vi "GrubbsTest_-_kopia.vi"() -> ()   [LabVIEW 2013]
uses:
  <vilib>/Analysis/NI_AALBase.lvlib
  <vilib>/Utility/file.llb/Read From Spreadsheet File (DBL).vi
panel:
  out "СКО":dbl
  out "Среднее":dbl
  out "Обработанные":dbl[](graph)
  out "Исходные":dbl[](graph)
  out "Промахи":dbl[](array[numeric])
  in  "Значимость":dbl
  in  "Path":path
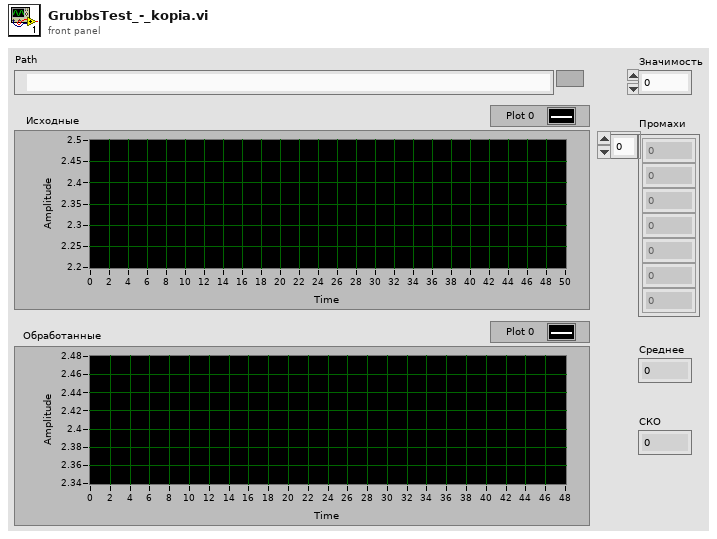
[diagram p1: front panel]
types:
  T1 = enum16{"Init", "GradeCount", "MissChecks", "fin"}
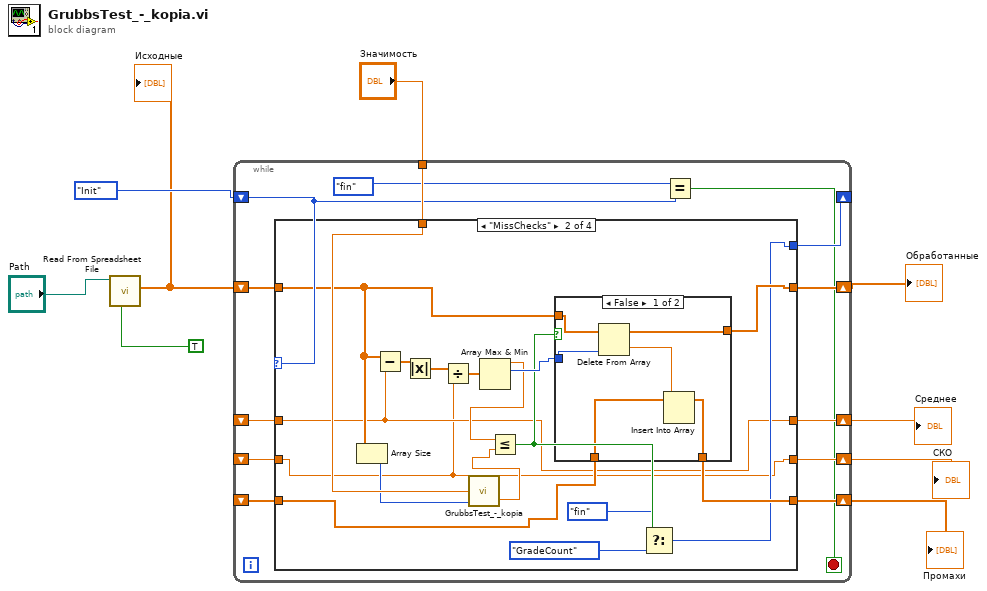
[diagram p0: block diagram]
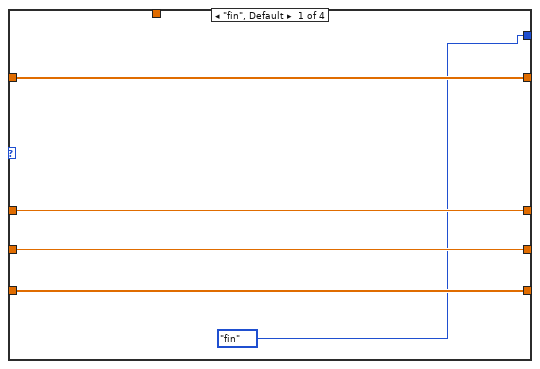
[diagram p2: hidden frame]
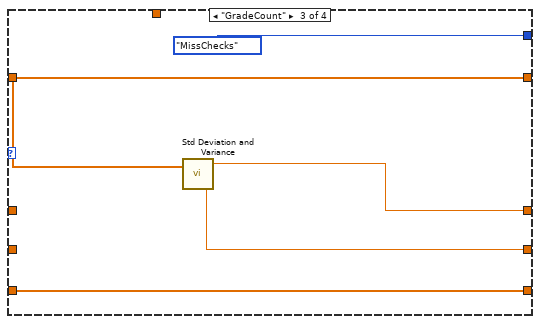
[diagram p4: hidden frame]
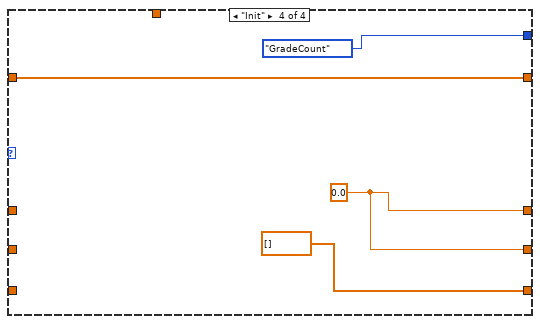
[diagram p5: hidden frame]
diagram:
  n1 = call-poly <vilib>:"Read From Spreadsheet File.vi"("transpose (no:F)"=TRUE, "file path (dialog if empty)"="Path") -> ("first row"=w7:dbl[])  [unwired: 5 in, 4 out]
  "Исходные" <- w7
  n2 = while {
    shift-right: [w22] -> _
    shift-left: T1."Init" -> [w11]
    tunnel: "Значимость" -> [w21]
    shift-right: [w16] -> w4
    shift-left: w7 -> [w20]
    shift-right: [w19] -> w3
    shift-left: _ -> [w13]
    shift-right: [w18] -> w2
    shift-left: _ -> [w14]
    shift-right: [w17] -> w1
    shift-left: _ -> [w15]
    stop <- w12 stop-if-true
    n3 = case shown="\"MissChecks\"" w11 {
      tunnel: [T1."fin" w34 T1."MissChecks" T1."GradeCount"] -> w22
      tunnel: w21 -> [_ w40 _ _]
      tunnel: w20 -> [w24 w31 w57 w61]
      tunnel: [w25 w30 w56 w60] -> w19
      tunnel: [w26 w29 w58 w60] -> w18
      tunnel: [w27 w44 w55 dbl[] []] -> w17
      tunnel: [w24 w43 w57 w61] -> w16
      tunnel: w15 -> [w27 w33 w55 _]
      tunnel: w14 -> [w26 w29 _ _]
      tunnel: w13 -> [w25 w30 _ _]
      frame "fin", Default {
      }
      frame "MissChecks" {
        n4 = Array Size(array=w31) -> (size(s)=w39:i32)
        n5 = Subtract(x=w31, y=w30) -> (x-y=w32:dbl[])
        n6 = Absolute Value(x=w32) -> (abs(x)=w45:dbl[])
        n7 = Divide(x=w45, y=w29) -> (x/y=w28:dbl[])
        n8 = call "GrubbsTest_-_kopia.vi"("n"=w39, "q"=w40) -> ("G"=w38:dbl)  [unwired: 2 in]
        n9 = Array Max & Min(array=w28) -> (max value=w41:dbl, max index (indices)=w42:i32)  [unwired: 2 out]
        n10 = Less Or Equal?(x=w41, y=w38) -> (x <= y?=w37:bool)
        n11 = case shown="False" w37 {
          tunnel: w31 -> [w50 w53]
          tunnel: [w47 w52] -> w44
          tunnel: [w49 w53] -> w43
          tunnel: w42 -> [w46 _]
          tunnel: w33 -> [w48 w52]
          frame False {
            n12 = Delete From Array(array=w50, index=w46) -> (deleted portion=w51:dbl, array with subset deleted=w49:dbl[])  [unwired: 1 in]
            n13 = Insert Into Array(array=w48, new element=w51) -> (w47:dbl[])  [unwired: 1 in]
          }
          frame True {
          }
        }
        n14 = Select(t=T1."fin", s=w37, f=T1."GradeCount") -> (s? t:f=w34:T1)
      }
      frame "GradeCount" {
        n15 = call <vilib>:"Std Deviation and Variance.vi"("X"=w57) -> ("mean"=w56:dbl, "standard deviation"=w58:dbl)  [unwired: 1 in, 1 out]
      }
      frame "Init" {
        w60 = 0.0
      }
    }
    n16 = Equal?(x=T1."fin", y=w11) -> (x = y?=w12:bool)
  }
  "Промахи" <- w1
  "Обработанные" <- w4
  "Среднее" <- w3
  "СКО" <- w2
